vi "Get Vehicle Parameters.vi"() -> ()   [LabVIEW 2019]
uses:
  VehicleType.ctl
  Car/Car.lvclass
  C:/Users/Kasia/Desktop/OOP/Solutions/Exercise 4/Vehicle/Vehicle.lvclass
  Car/Car.lvclass/Car.ctl
  Bicycle/Bicycle.lvclass
  Vehicle/Vehicle.lvclass/Vehicle.ctl
  Vehicle/Vehicle.lvclass
panel:
  in  "Horsepower":i32=130
  in  "Vehicle":T1
  out "Horsepower":i32
  out "Number of Wheels":i32
  out "Current Velocity":dbl
  # "SET"
  # "READ"
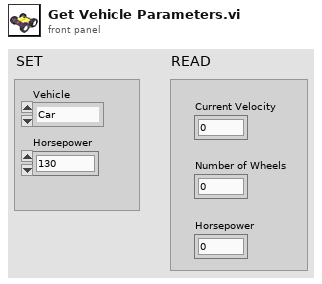
[diagram p1: front panel]
types:
  T1 = typedef "VehicleType.ctl" = enum16{"Car", "Bicycle"}
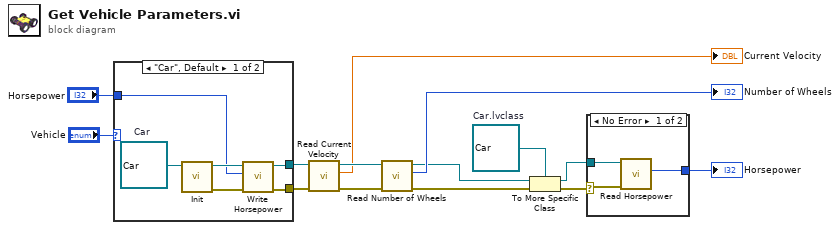
[diagram p0: block diagram]
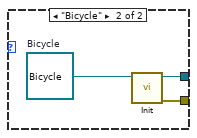
[diagram p2: hidden frame]
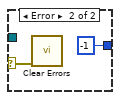
[diagram p3: hidden frame]
diagram:
  w9 = refnum<class "Car.lvclass"> refnum  # Car.lvclass
  n1 = case shown="\"Car\", Default" "Vehicle" {
    tunnel: [w18 w22] -> w3
    tunnel: [w17 w21] -> w2
    tunnel: "Horsepower" -> [w15 _]
    frame "Car", Default {
      w20 = refnum<class "Car.lvclass"> refnum  # Car
      n2 = call-dynamic "Init.vi"("Car in"=w20) -> ("error out"=w16:errorcluster, "Car out"=w19:refnum<class "Car.lvclass">)  [unwired: 9 in]
      n3 = call "Write Horsepower.vi"("error in (no error)"=w16, "Horsepower"=w15, "Car in"=w19) -> ("error out"=w17:errorcluster, "Car out"=w18:refnum<class "Car.lvclass">)  [unwired: 7 in]
    }
    frame "Bicycle" {
      w23 = refnum<class "Bicycle.lvclass"> refnum  # Bicycle
      n4 = call-dynamic "Init.vi"("Bicycle in"=w23) -> ("error out"=w21:errorcluster, "Bicycle out"=w22:refnum<class "Bicycle.lvclass">)  [unwired: 9 in]
    }
  }
  n5 = call "Read Current Velocity.vi"("error in (no error)"=w2, "Vehicle in"=w3) -> ("error out"=w13:errorcluster, "Current Velocity"=→"Current Velocity":dbl, "Vehicle out"=w14:refnum<class "Vehicle.lvclass">)  [unwired: 7 in]
  n6 = call "Read Number of Wheels .vi"("error in (no error)"=w13, "Vehicle in"=w14) -> ("error out"=w10:errorcluster, "Number of Wheels"=→"Number of Wheels":i32, "Vehicle out"=w5:refnum<class "Vehicle.lvclass">)  [unwired: 7 in]
  n7 = To More Specific Class(target class=w9, reference=w5, error in=w10) -> (specific class reference=w7:refnum<class "Car.lvclass">, error out=w8:errorcluster)
  n8 = case shown="No Error" w8 {
    selector: w8 -> [w25 w27]
    tunnel: w7 -> [w26 _]
    tunnel: [w24 -1 ("Horsepower")] -> w6
    frame No Error {
      n9 = call "Read Horsepower.vi"("error in (no error)"=w25, "Car in"=w26) -> ("Horsepower"=w24:i32)  [unwired: 7 in, 2 out]
    }
    frame Error {
      n10 = call <vilib>:"Clear Errors.vi"("error in (no error)"=w27) -> ()  [unwired: 5 in, 2 out]
    }
  }
  "Horsepower" <- w6
